vi "Running.vi"(8 "error in (no error)":errorcluster, 11 "CIFCorePlugin in":refnum<class "CIFCorePlugin.lvclass">) -> (0 "error out":errorcluster, 2 "Destroy":bool, 3 "CIFCorePlugin out":refnum<class "CIFCorePlugin.lvclass">)   [LabVIEW 2021, in "CIFCorePlugin.lvclass"]
uses:
  CIFCorePlugin.lvclass
  CIFCorePlugin.lvclass/CIFCorePlugin.ctl
  Channels/CIFChannelMng/CIFChannelMng.lvclass/CIFChannelMng.ctl
  CIFUtilities/CIFOutOfBand/CIFOutOfBand.lvclass/CIFOutOfBand.ctl
  Typedef/Energized States.ctl
  Accessors/Timestamps/Write Sleep TS.vi
  SubVIs/Read OOB RX.vi
  OOB/OOB_Tx/Send/Update Status Command.vi
  OOB/OOB_Tx/Send/Update Override Command.vi
  Accessors/Read Update Channel OOB.vi
  OOB/OOB_Tx/Send/Update Channel List Command.vi
  Accessors/Read Channel Status.vi
  Accessors/Write Update Channel OOB.vi
  CIFUtilities/CIFClocks/Core/Sleep Until Future Time.vi
  CIFUtilities/CIFClocks/Core/Get Time.vi
  Common/Utilities/Update Cycle Time.vi
  Common/Utilities/Update Delta Time.vi
  Accessors/Timestamps/Write Housekeeping TS.vi
  Benchmarking/Adjust Idle Benchmark.vi
  Accessors/Get Time.vi
  Accessors/Timestamps/Read Execute TS.vi
  Accessors/Timestamps/Read Housekeeping TS.vi
  Accessors/Timestamps/Read Sleep TS.vi
  Accessors/Timestamps/Read Target Wake TS.vi
  OOB/OOB_Rx/Receive/Check for OOB Commands.vi
  SubVIs/Refresh Stats.vi
  CIFUtilities/CIFOutOfBand/Write OOB DVR.vi
  CIFUtilities/CIFOutOfBand/Utilities/Command to Bitwise Command.vi
  CIFUtilities/CIFOutOfBand/Accessors/Read Local OOB Data.vi
  CIFUtilities/CIFOutOfBand/Accessors/Write Local OOB Data.vi
  Channels/CIFChannelMng/Accessors/Read Update OOB.vi
  Channels/CIFChannelMng/Accessors/Read Channel Status for OOB.vi
  Channels/CIFChannelMng/Accessors/Write Update OOB.vi
  CIFUtilities/CIFClocks/SubVIs/Add Error.vi
  CIFUtilities/CIFClocks/Time Conversion/LabVIEW Time to UTC Time.vi
  CIFUtilities/CIFOutOfBand/Read OOB DVR.vi
  OOB/OOB_Rx/Private/Command Settings.vi
  Common/Utilities/Append Error Location.vi
  OOB/OOB_Tx/CIFCoreOOB_Tx.lvclass
  D:/dev/CIF-LVCore/src/CIFUtilities/CIFOutOfBand/CIFOutOfBand.lvclass
  OOB/OOB_Rx/CIFCoreOOB_Rx.lvclass
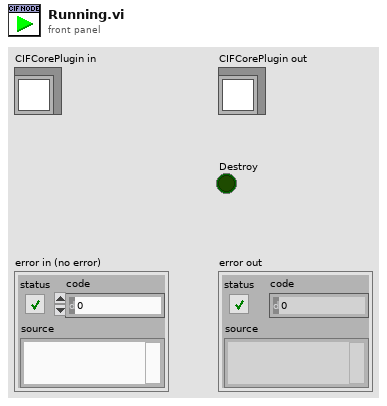
[diagram p1: front panel]
types:
  T1 = typedef "CIFCorePlugin.lvclass/Energized States.ctl" = enum16{"Listen", "Prepare", "Execute", "Housekeep", "Cleanup", "Destroy"}
  T2 = typedef "CIFCorePlugin.lvclass/Running State Logic.ctl" = enum16{"Execute", "Housekeep", "Cleanup", "Error", "Destroy"}
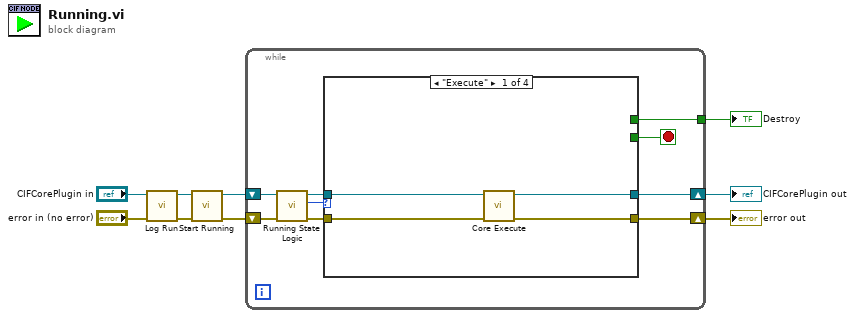
[diagram p0: block diagram]
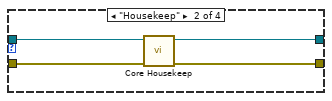
[diagram p2: hidden frame]
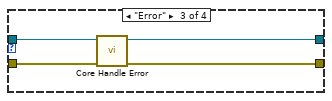
[diagram p3: hidden frame]
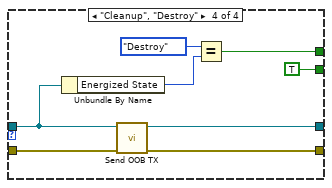
[diagram p4: hidden frame]
diagram:
  n1 = call "Log Run.vi"("error in (no error)"="error in (no error)", "CIFCorePlugin in"="CIFCorePlugin in") -> ("error out"=w2:errorcluster, "CIFCorePlugin out"=w1:refnum<class "CIFCorePlugin.lvclass">)  [unwired: 8 in]
  n2 = call "Start Running.vi"("error in (no error)"=w2, "CIFCorePlugin in"=w1) -> ("error out"=w5:errorcluster, "CIFCorePlugin out"=w6:refnum<class "CIFCorePlugin.lvclass">)  [unwired: 8 in]
  n3 = while {
    shift-right: [w13] -> w8
    shift-left: w6 -> [w18]
    shift-right: [w12] -> w7
    shift-left: w5 -> [w17]
    tunnel: [w10] -> w9
    stop <- w11 stop-if-true
    n4 = call "Running State Logic.vi"("error in (no error)"=w17, "CIFCorePlugin in"=w18) -> ("error out"=w14:errorcluster, "Running State Logic"=w16:T2, "CIFCorePlugin out"=w15:refnum<class "CIFCorePlugin.lvclass">)  [unwired: 7 in]
    n5 = case shown="\"Execute\"" w16 {
      tunnel: w15 -> [w21 w26 w30 w34]
      tunnel: w14 -> [w22 w25 w29 w37]
      tunnel: [w19 w24 w28 w36] -> w13
      tunnel: [w20 w23 w27 w35] -> w12
      tunnel: [_ _ _ TRUE] -> w11
      tunnel: [_ _ _ w31] -> w10
      frame "Execute" {
        n6 = call "Core Execute.vi"("error in (no error)"=w22, "CIFTemplateNode in"=w21) -> ("error out"=w20:errorcluster, "CIFTemplateNode out"=w19:refnum<class "CIFCorePlugin.lvclass">)  [unwired: 8 in]
      }
      frame "Housekeep" {
        n7 = call "Core Housekeep.vi"("error in (no error)"=w25, "CIFCorePlugin in"=w26) -> ("error out"=w23:errorcluster, "CIFCorePlugin out"=w24:refnum<class "CIFCorePlugin.lvclass">)  [unwired: 8 in]
      }
      frame "Error" {
        n8 = call "Core Handle Error.vi"("error in (no error)"=w29, "CIFTemplateNode in"=w30) -> ("error out"=w27:errorcluster, "CIFTemplateNode out"=w28:refnum<class "CIFCorePlugin.lvclass">)  [unwired: 8 in]
      }
      frame "Cleanup", "Destroy" {
        n9 = Unbundle By Name(w34) -> ("Energized State"=w33:T1)
        n10 = call "Send OOB TX.vi"("error in (no error)"=w37, "CIFCorePlugin in"=w34) -> ("error out"=w35:errorcluster, "CIFCorePlugin out"=w36:refnum<class "CIFCorePlugin.lvclass">)  [unwired: 8 in]
        n11 = Equal?(x=Energized_States."Destroy", y=w33) -> (x = y?=w31:bool)
      }
    }
  }
  "error out" <- w7
  "CIFCorePlugin out" <- w8
  "Destroy" <- w9
